vi "ReadYourSuggestion.vi"() -> ()   [LabVIEW 2023]
uses:
  <vilib>/Utility/file.llb/Read Delimited Spreadsheet (DBL).vi
panel:
  out "appended array":u64[][][](array[numeric])
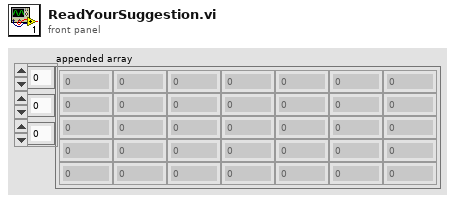
[diagram p1: front panel]
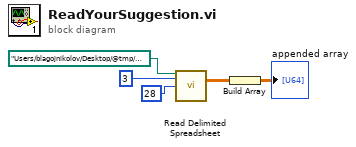
[diagram p0: block diagram]
diagram:
  n1 = call-poly <vilib>:"Read Delimited Spreadsheet.vi"("file path (dialog if empty)"=path "/Users/blagojnikolov/Desktop/@tmp/toto.txt", "number of rows (all:-1)"=3 ("start of read offset (chars.:0)"), "start of read offset (chars.:0)"=28) -> ("all rows"=w4:dbl[][])  [unwired: 7 in, 5 out]
  n2 = Build Array(w4) -> (→"appended array":dbl[][][])
